vi "AH2700_write_data.vi"(7 "File reference":refnum<file>) -> ()   [LabVIEW 2019]
uses:
  Global/Global Variables/Data_Display_global.vi
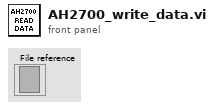
[diagram p1: front panel]
types:
  T1 = typedef "AH2700-Cluster.ctl" = cluster{"Units Display":i32, "Sample Switch":i32, "Frequency":dbl, "V excitation":dbl, "Capacity Graphic":dbl[][], "Loss Graphic":dbl[][], "Capacity":dbl, "Loss":dbl, "Update AH2500":bool, "Bias ":dbl, " AVerage":dbl}
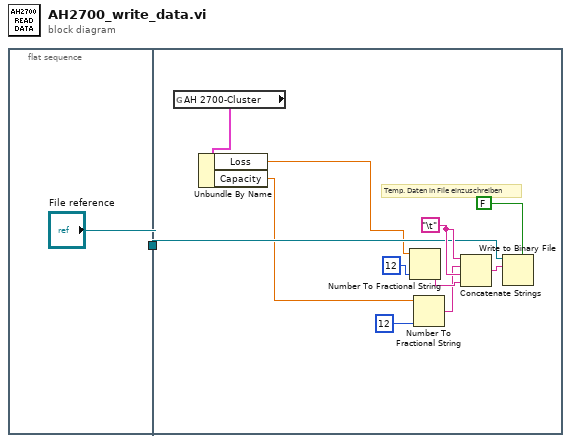
[diagram p0: block diagram]
diagram:
  n1 = flat-sequence {
    tunnel: ["File reference"] -> w1
    tunnel: w1 -> [w6]
    frame #0 {
    }
    frame #1 {
      w11 = "\t"
      # "Temp. Daten in File einzuschreiben"
      n2 = global read "Data_Display_global.vi" "AH 2700-Cluster"() -> (w5:T1)
      n3 = Unbundle By Name(w5) -> ("Loss"=w4:dbl, "Capacity"=w3:dbl)
      n4 = Number To Fractional String(number=w4, precision (6)=i16 12) -> (F-format string=w12:string)  [unwired: 2 in]
      n5 = Number To Fractional String(number=w3, precision (6)=i16 12) -> (F-format string=w8:string)  [unwired: 2 in]
      n6 = Concatenate Strings(w11, w8, w11, w12) -> (w13:string)
      n7 = Write to Binary File ("Write File")(file (use dialog)=w6, data=w13, 5:FALSE ("prepend array or string size? (T)")) -> ()  [unwired: 3 in, 3 out]
    }
  }
